vi "SetCurrent.vi"(3 "Current":u16 step=1, 4 "error in":errorcluster, 5 "connection ID in":refnum<k5>) -> (0 "False":bool, 1 "error out":errorcluster, 2 "connection ID out":refnum<k5>)   [LabVIEW 2015]
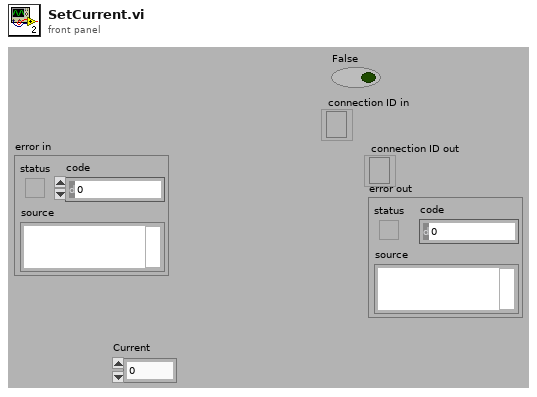
[diagram p1: front panel]
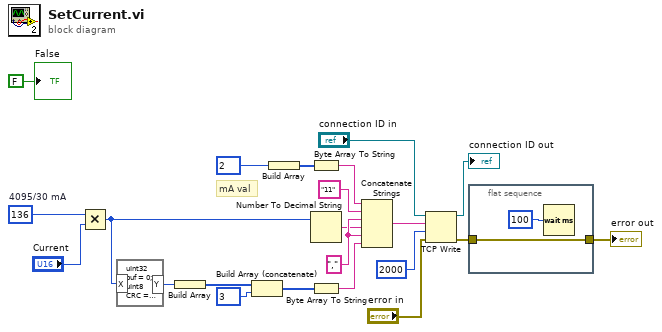
[diagram p0: block diagram]
diagram:
  w7 = u16 136  # 4095/30 mA
  w12 = "," ("string")
  # "mA val"
  n1 = Multiply(x=w7, y="Current") -> (x*y=w1:u16)
  n2 = formula code="uInt32 buf = 0;\nuInt8 CRC = 0;\nuInt8 Y = 0;\n\nbuf = 0x31 + 0x31  + X + 0x2C;\nbuf = ~ buf;\nbuf = buf & 0x000000FF;\nCRC = buf;\nCRC &= 0x7F;\nCRC |= 0x40;\nCRC++;\nY = CRC;"("X"=w1) -> ("Y"=w11:u8)
  n3 = Build Array(w11) -> (w10:u8[])
  n4 = Build Array (concatenate)(w10, u8 3 ("y")) -> (w17:u8[])
  n5 = Build Array(u8 2 ("y")) -> (w15:u8[])
  n6 = Byte Array To String(unsigned byte array=w15) -> (string=w14:string)
  n7 = Number To Decimal String(number=w1) -> (decimal integer string=w8:string)  [unwired: 1 in]
  n8 = Byte Array To String(unsigned byte array=w17) -> (string=w9:string)
  n9 = Concatenate Strings(w14, "11" ("string"), w12, w8, w12, w9) -> (w5:string)
  n10 = TCP Write(connection ID="connection ID in", data in=w5, error in (no error)="error in", 9:2000 ("timeout ms (25000)")) -> (connection ID out=→"connection ID out":refnum<k5>, error out=w3:errorcluster)  [unwired: 1 out]
  n11 = flat-sequence {
    tunnel: [w24] -> w2
    tunnel: w3 -> [w24]
    frame #0 {
      n12 = Wait (ms)(milliseconds to wait=u32 100) -> ()  [unwired: 1 out]
    }
  }
  "error out" <- w2
  "False" <- FALSE
